vi "read entry.vi"(8 "error in (no error)":errorcluster, 11 "id":string) -> (0 "error out":errorcluster, 3 "entry":T1)   [LabVIEW 2024, in "status manager.lvlib"]
uses:
  status manager.lvlib
  entry type.ctl
  fgv actions.ctl
  <vilib>/Utility/error.llb/Error Cluster From Error Code.vi
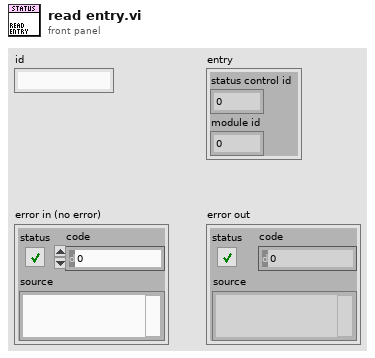
[diagram p1: front panel]
types:
  T1 = typedef "status manager.lvlib/entry type.ctl" = cluster{"status control id":i32, "module id":i32}
  T2 = typedef "status manager.lvlib/fgv actions.ctl" = enum16{"create", "get", "destroy"}
  T3 = typedef "status manager.lvlib/collection type.ctl" = map{string, T1}
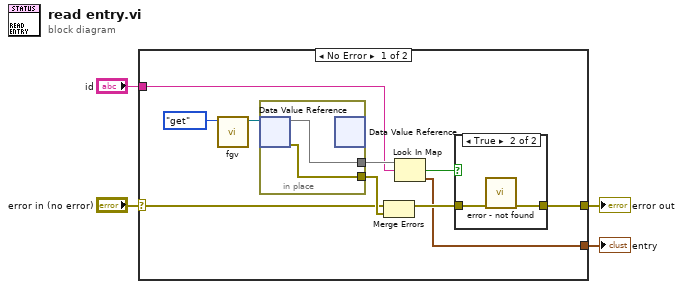
[diagram p0: block diagram]
diagram:
  n1 = case shown="No Error" "error in (no error)" {
    selector: "error in (no error)" -> [w11 w20]
    tunnel: [w6 w20] -> w3
    tunnel: "id" -> [w9 _]
    tunnel: [w5 _] -> w1
    frame No Error {
      n2 = call "fgv.vi"("action"=fgv_actions."get") -> ("dvr"=w14:refnum<data-value>)  [unwired: 9 in, 1 out]
      n3 = in-place {
        in-place-border: [w19] -> w10
        in-place-border: [w18] -> w12
        n4 = in-place-dvr #1(w14) -> (w19:T3, w18:errorcluster)
        n5 = in-place-dvr #1() -> ()  [unwired: 1 in, 2 out]
      }
      n6 = Merge Errors(w11, w12) -> (w7:errorcluster)
      n7 = Look In Map(map=w10, key=w9) -> (key not found?=w8:bool, value=w5:T1)  [unwired: 1 in]
      n8 = case shown="True" w8 {
        tunnel: w7 -> [w15 w17]
        tunnel: [w15 w16] -> w6
        frame False {
        }
        frame True {
          n9 = call "error - not found.vi"("error in (no error)"=w17) -> ("error out"=w16:errorcluster)  [unwired: 10 in]
        }
      }
    }
    frame Error {
    }
  }
  "error out" <- w3
  "entry" <- w1
